vi "Coordinate_Outlier_Filtering_R2.vi"(0 "Num of Beacons":i8=5, 1 "Max Std Dev(all 5)":dbl=1.0, 5 "X in":sgl[](array[numeric]), 7 "Valid Data\nSets in":bool[](array[boolean])=[TRUE, TRUE, TRUE, TRUE, TRUE], 9 "Y in":sgl[](array[numeric]), 11 "Max Std Dev( 4 )":dbl=1.0, 13 "Max Std Dev (3)":dbl=1.0) -> (3 "Y out":sgl[](array[numeric]), 4 "Max":i32, 6 "Min Std Dev\nfor Max beacons":dbl, 8 "X out":sgl[](array[numeric]), 10 "Valid Beacons\nout":bool[](array[boolean]), 15 "Slope out":dbl)   [LabVIEW 2015]
uses:
  <vilib>/Analysis/NI_AALPro.lvlib
panel:
  out "std dev_current":dbl format="%0.6f"
  out "std dev_current 3":dbl format="%0.6f"
  out "size(s) 2":i32
  out "std dev_current 2":dbl format="%0.6f"
  out "size(s)":i32
  in  "Combo_info\nTemplate":T1={"Num Beacons"=0, "Std Dev_combo"=0.0, "Valid Data\nSets_combo"=[FALSE, FALSE, FALSE, FALSE, FALSE], "Slope combo"=0.0}
types:
  T1 = cluster{"Num Beacons":u8, "Std Dev_combo":dbl, "Valid Data\nSets_combo":bool[], "Slope combo":dbl}
  T2 = cluster{"dimension size":u8, sgl, bool[], "slope":dbl}
  T3 = cluster{"dimension size":u8, "Std Dev_combo":dbl, "Valid Data\nSets_combo":bool[], "slope":dbl}[]
  T4 = cluster{"dimension size":u8, dbl, bool[], "slope":dbl}
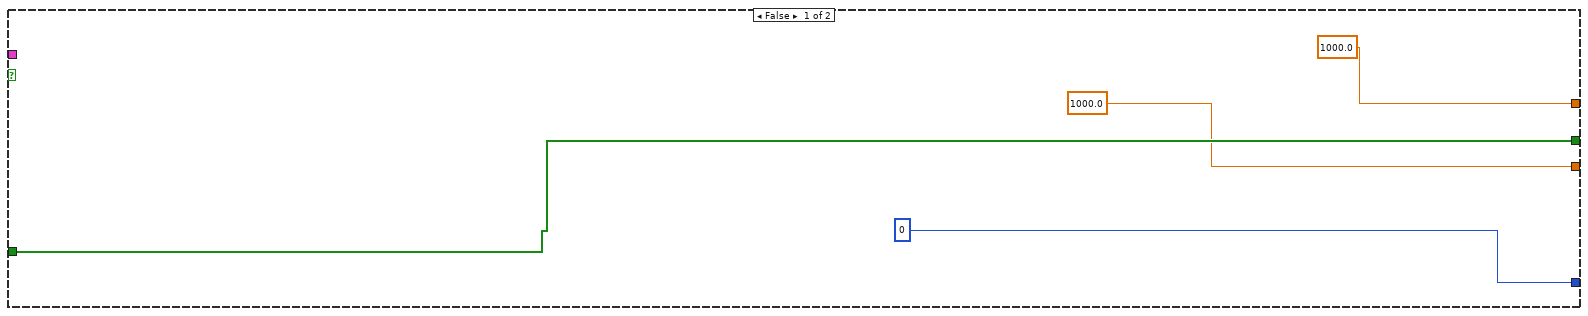
[diagram p5: hidden frame]
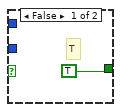
[diagram p10: hidden frame]
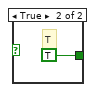
[diagram p11: hidden frame]
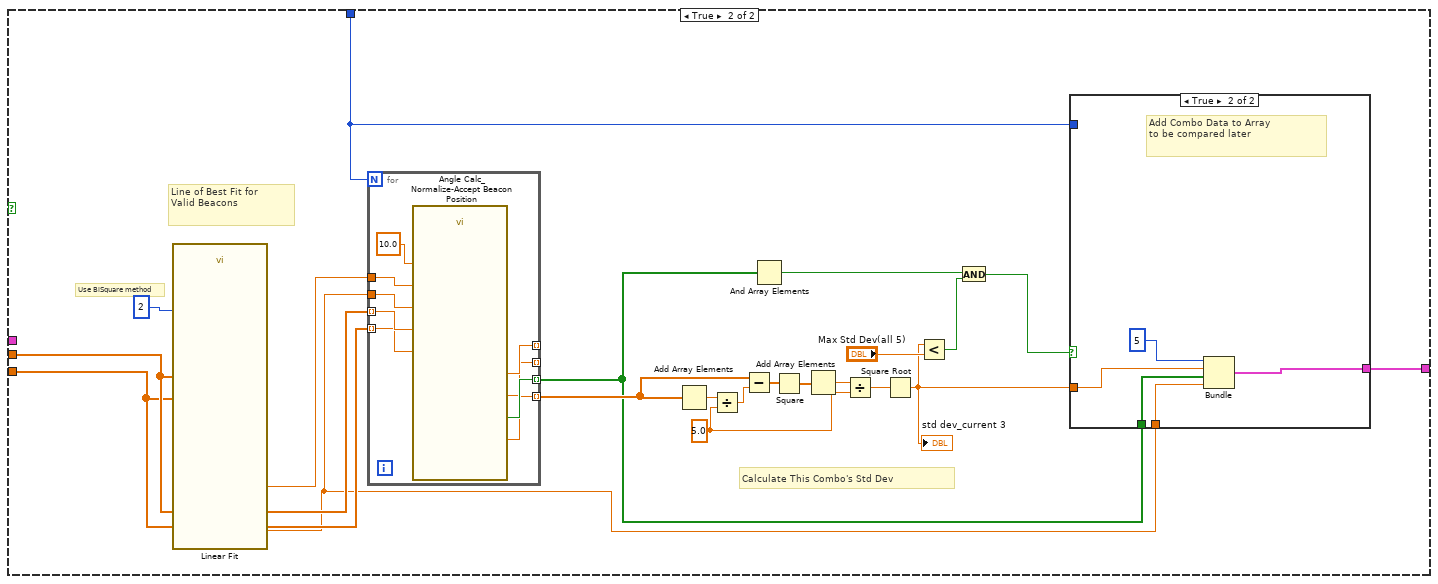
[diagram p15: hidden frame]
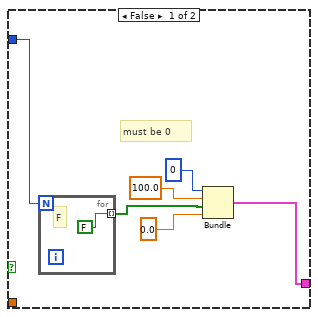
[diagram p16: hidden frame]
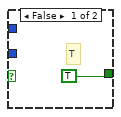
[diagram p18: hidden frame]
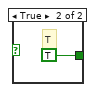
[diagram p19: hidden frame]
diagram:
  w2 = i16 2 ("y")
  # "Use BiSquare method"
  # "Line of Best Fit for\nValid Beacons"
  n1 = Boolean To (0,1)(Boolean="Valid Data\nSets in") -> (0, 1=w21:i16[])
  n2 = Add Array Elements(numeric array=w21) -> (sum=w3:i16)
  n3 = Greater?(x=w3, y=w2) -> (0:w4:bool)
  n4 = case shown="False" w4 {
    tunnel: "Combo_info\nTemplate" -> [_ w92]
    tunnel: w3 -> [_ w87]
    tunnel: "Valid Data\nSets in" -> [w24 w86]
    tunnel: [0.0 w80] -> w18
    tunnel: [0 w79] -> w17
    tunnel: [w23 w75] -> w16
    tunnel: "X in" -> [w26 w74]
    tunnel: "Y in" -> [w25 w73]
    tunnel: [w24 w72] -> w6
    tunnel: "Num of Beacons" -> [w32 w70]
    tunnel: w2 -> [w31 _]
    frame False {
      # "Use BiSquare method"
      # "Line of Best Fit for\nValid Beacons"
      # "Average"
      n5 = disable-structure shown="Disabled" {
        disable-tunnel: w26 -> [w43 _]
        disable-tunnel: w25 -> [w42 _]
        disable-tunnel: w24 -> [w41 _]
        disable-tunnel: w32 -> [w35 _]
        disable-tunnel: w31 -> [w34 _]
        frame Disabled {
          # "Grab the 2 valid coordinates"
          n6 = Initialize Array(sgl 0.0, w34) -> (w37:sgl[])
          n7 = Initialize Array(sgl 0.0, w34) -> (w38:sgl[])
          n8 = while {
            tunnel: w43 -> [w55] mode=indexing
            tunnel: w42 -> [w54] mode=indexing
            tunnel: w41 -> [w58] mode=indexing
            shift-right: [w50] -> _
            shift-left: i16 0 ("y") -> [w57]
            shift-right: [w52] -> _
            shift-left: w38 -> [w56]
            shift-right: [w51] -> _
            shift-left: w37 -> [w53]
            tunnel: w35 -> [w45]
            tunnel: w34 -> [w44]
            i -> [w46]
            stop <- w49 stop-if-true
            n9 = case shown="True" w58 {
              tunnel: w57 -> [w61 w65]
              tunnel: w56 -> [w60 w68]
              tunnel: [w61 w69] -> w50
              tunnel: w55 -> [_ w67]
              tunnel: w54 -> [_ w64]
              tunnel: w53 -> [w59 w66]
              tunnel: [w60 w63] -> w52
              tunnel: [w59 w62] -> w51
              frame False {
              }
              frame True {
                n10 = Replace Array Subset(array=w68, new element=w67, index=w65) -> (w63:sgl[])
                n11 = Replace Array Subset(array=w66, new element=w64, index=w65) -> (w62:sgl[])
                n12 = Increment(x=w65) -> (x+1=w69:i16)
              }
            }
            n13 = Greater Or Equal?(x=w46, y=w45) -> (x >= y?=w47:bool)
            n14 = Greater Or Equal?(x=w50, y=w44) -> (x >= y?=w48:bool)
            n15 = Or(x=w48, y=w47) -> (x .or. y?=w49:bool)
          }
        }
        frame Enabled {
        }
      }
      n16 = Boolean To (0,1)(Boolean=w24) -> (0, 1=w28:i16[])
      n17 = Add(x=w28, y=1e-12) -> (x+y=w30:dbl[])
      n18 = call <vilib>:"Linear Fit.vi"("Y"=w25, "X"=w26, "Weight"=w30, "method"=2) -> ("slope"=w23:dbl)  [unwired: 7 in, 4 out]
    }
    frame True {
      # "5  Beacon Combination (only 1)"
      # "4 Beacon Combinations"
      # "3 Beacon Combinations"
      n19 = Equal?(x=w87, y=5 ("dimension size")) -> (x = y?=w95:bool)
      n20 = case shown="False" w95 {
        tunnel: w74 -> [_ w320]
        tunnel: w73 -> [_ w319]
        tunnel: w70 -> [_ w304]
        tunnel: [w301 w305] -> w93
        tunnel: w92 -> [w301 _]
        frame False {
        }
        frame True {
          w303 = sgl 5.0 ("y")
          # "Calculate This Combo's Std Dev"
          # "Use BiSquare method"
          # "Line of Best Fit for\nValid Beacons"
          n21 = call <vilib>:"Linear Fit.vi"("Y"=w319, "X"=w320, "method"=2) -> ("slope"=w302:dbl, "intercept"=w321:dbl)  [unwired: 8 in, 3 out]
          n22 = for {
            N: w304 -> [_]
            tunnel: w302 -> [w342]
            tunnel: w321 -> [w341]
            tunnel: w320 -> [w340] mode=indexing
            tunnel: w319 -> [w339] mode=indexing
            tunnel: [w338] -> w306 mode=indexing
            tunnel: [w337] -> w307 mode=indexing
            tunnel: [w336] -> _ mode=indexing
            tunnel: [w335] -> _ mode=indexing
            n23 = call "Angle Calc_Normalize-Accept Beacon Position.vi"("slope"=w342, "Xin"=w340, "Deviation Threshold"=sgl 10.0 ("Deviation Threshold\n- Local Beacon Pos(*unit)"), "intercept"=w341, "Yin"=w339) -> ("Accept Beacon"=w338:bool, "Xout"=w336:sgl, "Distance"=w337:sgl, "Yout"=w335:sgl)  [unwired: 6 in, 1 out]
          }
          n24 = Add Array Elements(numeric array=w307) -> (sum=w318:sgl)
          n25 = Divide(x=w318, y=w303) -> (x/y=w317:sgl)
          n26 = Subtract(x=w307, y=w317) -> (x-y=w316:sgl[])
          n27 = And Array Elements(Boolean array=w306) -> (logical AND=w312:bool)
          n28 = Square(x=w316) -> (x^2=w308:sgl[])
          n29 = Add Array Elements(numeric array=w308) -> (sum=w314:sgl)
          n30 = Divide(x=w314, y=w303) -> (x/y=w315:sgl)
          n31 = Square Root(x=w315) -> (sqrt(x)=w310:sgl)
          "std dev_current 3" <- w310
          n32 = Less?(x=w310, y="Max Std Dev(all 5)") -> (x < y?=w311:bool)
          n33 = And(x=w312, y=w311) -> (x .and. y?=w309:bool)
          n34 = case shown="True" w309 {
            tunnel: w310 -> [_ w333]
            tunnel: w306 -> [_ w332]
            tunnel: [w325 w331] -> w305
            tunnel: w304 -> [w324 _]
            tunnel: w302 -> [_ w330]
            frame False {
              # "must be 0"
              n35 = for {
                N: w324 -> [_]
                tunnel: [FALSE] -> w326 mode=indexing
                # "F"
              }
              n36 = Bundle("dimension size"=u8 0, 100.0, w326, 0.0) -> (w325:cluster{"dimension size":u8, dbl, bool[], dbl})  [unwired: 1 in]
            }
            frame True {
              # "Add Combo Data to Array\nto be compared later"
              n37 = Bundle("dimension size"=u8 5, w333, w332, "slope"=w330) -> (w331:T2)  [unwired: 1 in]
            }
          }
        }
      }
      n38 = Build Array(w93) -> (w91:T3)
      n39 = Greater Or Equal?(x=w87, y=i16 4) -> (x >= y?=w98:bool)
      n40 = case shown="True" w98 {
        tunnel: w70 -> [_ w348]
        tunnel: w74 -> [_ w351]
        tunnel: w73 -> [_ w350]
        tunnel: w86 -> [_ w349]
        tunnel: w91 -> [w344 w347]
        tunnel: [w344 w346] -> w90
        tunnel: w70 -> [_ w345]
        frame False {
        }
        frame True {
          n41 = for {
            N: w348 -> [w355]
            shift-right: [w353] -> w346
            shift-left: w347 -> [w354]
            tunnel: w351 -> [w358]
            tunnel: w350 -> [w357]
            tunnel: w349 -> [w359]
            tunnel: w345 -> [w352]
            i -> [w356]
            n42 = for {
              N: w355 -> [w363]
              tunnel: w356 -> [w365]
              shift-right: [w361] -> w353
              shift-left: w354 -> [w362]
              tunnel: w358 -> [w367]
              tunnel: w357 -> [w366]
              tunnel: w359 -> [w368]
              tunnel: w352 -> [w360]
              i -> [w364]
              n43 = for {
                N: w363 -> [w371]
                tunnel: w368 -> [w377]
                tunnel: w367 -> [w376]
                tunnel: w366 -> [w375]
                tunnel: w365 -> [w372]
                tunnel: w364 -> [w378]
                shift-right: [w374] -> w361
                shift-left: w362 -> [w370]
                tunnel: w360 -> [w369]
                i -> [w373]
                n44 = for {
                  N: w371 -> [w388]
                  tunnel: w378 -> [w390]
                  tunnel: w377 -> [w413]
                  tunnel: w376 -> [w411]
                  tunnel: w375 -> [w410]
                  tunnel: w373 -> [w391]
                  tunnel: w372 -> [w389]
                  shift-right: [w400] -> w374
                  shift-left: w370 -> [w392]
                  tunnel: w369 -> [w379]
                  i -> [w387]
                  w393 = 4
                  # "Build Beacon Set Boolean Array\n(correlates to indexes)"
                  # "Fetch Coordinates"
                  # "Are All Indexes Different?\nAND\nDo those indexes contain valid beacons?\nAND\nIs it not a repeat combo?"
                  n45 = Greater?(x=w391, y=w390) -> (0:w383:bool)
                  n46 = Greater?(x=w390, y=w389) -> (0:w384:bool)
                  n47 = Greater?(x=w387, y=w391) -> (0:w382:bool)
                  n48 = Build Array(w389, w390, w391, w387) -> (w398:i32[])
                  n49 = for {
                    N: w393 -> [_]
                    tunnel: w398 -> [w417] mode=indexing
                    tunnel: w398 -> [w418]
                    tunnel: [w415] -> w397 mode=indexing
                    tunnel: w393 -> [w414]
                    i -> [w419]
                    n50 = for {
                      N: w414 -> [_]
                      tunnel: w419 -> [w424]
                      tunnel: w418 -> [w422] mode=indexing
                      tunnel: w417 -> [w421]
                      tunnel: [w420] -> w416 mode=indexing
                      i -> [w423]
                      n51 = Not Equal?(x=w424, y=w423) -> (x != y?=w425:bool)
                      n52 = case shown="True" w425 {
                        tunnel: w422 -> [_ w428]
                        tunnel: w421 -> [_ w427]
                        tunnel: [TRUE w429] -> w420
                        frame False {
                          # "T"
                        }
                        frame True {
                          n53 = Not Equal?(x=w427, y=w428) -> (x != y?=w429:bool)
                        }
                      }
                    }
                    n54 = And Array Elements(Boolean array=w416) -> (logical AND=w415:bool)
                  }
                  n55 = And Array Elements(Boolean array=w397) -> (logical AND=w381:bool)
                  n56 = Index Array(array=w411, index #1=w389, index #2=w390, index #3=w391, index #4=w387) -> (element #1=w409:sgl, element #2=w408:sgl, element #3=w407:sgl, element #4=w386:sgl)
                  n57 = Index Array(array=w410, index #1=w389, index #2=w390, index #3=w391, index #4=w387) -> (element #1=w406:sgl, element #2=w405:sgl, element #3=w404:sgl, element #4=w385:sgl)
                  n58 = Index Array(array=w413, index #1=w389, index #2=w390, index #3=w391, index #4=w387) -> (element #1=w396:bool, element #2=w395:bool, element #3=w394:bool, element #4=w380:bool)
                  n59 = for {
                    N: w388 -> [_]
                    tunnel: w391 -> [w440]
                    tunnel: w390 -> [w439]
                    tunnel: w389 -> [w438]
                    tunnel: [w433] -> w399 mode=indexing
                    tunnel: w387 -> [w431]
                    i -> [w432]
                    n60 = Equal?(x=w438, y=w432) -> (x = y?=w435:bool)
                    n61 = Equal?(x=w440, y=w432) -> (x = y?=w437:bool)
                    n62 = Equal?(x=w439, y=w432) -> (x = y?=w436:bool)
                    n63 = Equal?(x=w431, y=w432) -> (x = y?=w430:bool)
                    n64 = Compound Arithmetic op=OR(w437, w436, w435, w430) -> (w434:bool)
                    n65 = case shown="False" w434 {
                      tunnel: [FALSE TRUE] -> w433
                      frame False {
                        # "F"
                      }
                      frame True {
                        # "T"
                      }
                    }
                  }
                  n66 = Build Array(w409, w408, w407, w386) -> (w403:sgl[])
                  n67 = Build Array(w406, w405, w404, w385) -> (w402:sgl[])
                  n68 = Build Array(w396, w395, w394, w380) -> (w401:bool[])
                  n69 = Compound Arithmetic op=AND(w396, w395, w394, w380, w381, w382, w383, w384) -> (w412:bool)
                  n70 = case shown="True" w412 {
                    tunnel: w403 -> [_ w461]
                    tunnel: w402 -> [_ w462]
                    tunnel: w401 -> [_ w452]
                    tunnel: w392 -> [w443 w450]
                    tunnel: [w443 w448] -> w400
                    tunnel: w399 -> [_ w446]
                    tunnel: w379 -> [_ w445]
                    frame False {
                    }
                    frame True {
                      # "Calculate Distance from\nBeacon to Fitted Line"
                      # "Calculate This Combo's Std Dev"
                      # "Trim Arrays to Only Valid Beacons"
                      # "Use BiSquare method"
                      # "Line of Best Fit for\nValid Beacons"
                      # "All Indexes are Different and Beacons are Valid"
                      n71 = Initialize Array(sgl 0.0 ("element"), 4 ("dimension size")) -> (w470:sgl[])
                      n72 = for {
                        N: w445 -> [_]
                        shift-right: [w489] -> w459
                        shift-left: 0.0 -> [w490]
                        shift-right: [w488] -> w464
                        shift-left: w470 -> [w487]
                        shift-right: [w485] -> w463
                        shift-left: w470 -> [w486]
                        tunnel: w452 -> [w484] mode=indexing
                        tunnel: w461 -> [w483] mode=indexing
                        tunnel: w462 -> [w482] mode=indexing
                        n73 = case shown="True" w484 {
                          tunnel: w490 -> [w493 w500]
                          tunnel: [w493 w501] -> w489
                          tunnel: [w492 w498] -> w488
                          tunnel: w487 -> [w492 w497]
                          tunnel: w486 -> [w491 w496]
                          tunnel: [w491 w499] -> w485
                          tunnel: w483 -> [_ w495]
                          tunnel: w482 -> [_ w494]
                          frame False {
                          }
                          frame True {
                            n74 = Replace Array Subset(array=w497, new element=w495, index=w500) -> (w498:sgl[])
                            n75 = Replace Array Subset(array=w496, new element=w494, index=w500) -> (w499:sgl[])
                            n76 = Increment(x=w500) -> (x+1=w501:dbl)
                          }
                        }
                      }
                      n77 = call <vilib>:"Linear Fit.vi"("Y"=w463, "X"=w464, "method"=2) -> ("slope"=w444:dbl, "intercept"=w472:dbl)  [unwired: 8 in, 3 out]
                      n78 = for {
                        N: w445 -> [_]
                        tunnel: w472 -> [w510]
                        tunnel: w444 -> [w509]
                        tunnel: w464 -> [w508] mode=indexing
                        tunnel: w463 -> [w507] mode=indexing
                        tunnel: [w506] -> w455 mode=indexing
                        tunnel: [w505] -> _ mode=indexing
                        tunnel: [w504] -> _ mode=indexing
                        tunnel: [w503] -> w457 mode=indexing
                        n79 = call "Angle Calc_Normalize-Accept Beacon Position.vi"("slope"=w509, "Xin"=w508, "Deviation Threshold"=sgl 10.0 ("Deviation Threshold\n- Local Beacon Pos(*unit)"), "intercept"=w510, "Yin"=w507) -> ("Accept Beacon"=w506:bool, "Xout"=w505:sgl, "Distance"=w503:sgl, "Yout"=w504:sgl)  [unwired: 6 in, 1 out]
                      }
                      n80 = Add Array Elements(numeric array=w457) -> (sum=w469:sgl)
                      n81 = Divide(x=w469, y=w459) -> (x/y=w468:dbl)
                      n82 = Subtract(x=w457, y=w468) -> (x-y=w467:dbl[])
                      n83 = And Array Elements(Boolean array=w455) -> (logical AND=w454:bool)
                      n84 = Square(x=w467) -> (x^2=w456:dbl[])
                      n85 = Add Array Elements(numeric array=w456) -> (sum=w465:dbl)
                      n86 = Divide(x=w465, y=w459) -> (x/y=w466:dbl)
                      n87 = Square Root(x=w466) -> (sqrt(x)=w451:dbl)
                      "std dev_current 2" <- w451
                      n88 = Less?(x=w451, y="Max Std Dev( 4 )") -> (x < y?=w453:bool)
                      n89 = And(x=w454, y=w453) -> (x .and. y?=w449:bool)
                      n90 = case shown="True" w449 {
                        tunnel: w446 -> [_ w481]
                        tunnel: w451 -> [_ w480]
                        tunnel: w450 -> [w474 w479]
                        tunnel: [w474 w478] -> w448
                        tunnel: w444 -> [_ w475]
                        frame False {
                        }
                        frame True {
                          # "Add Combo Data to Array\nto be compared later"
                          n91 = Bundle("dimension size"=u8 4, w480, w481, "slope"=w475) -> (w476:T4)  [unwired: 1 in]
                          n92 = Build Array (concatenate)(w479, w476) -> (w478:T3)
                        }
                      }
                    }
                  }
                }
              }
            }
          }
        }
      }
      n93 = Array Size(array=w90) -> (size(s)=w96:i32)
      n94 = Decrement(x=w96) -> (x-1=w85:i32)
      "size(s) 2" <- w85
      n95 = Greater Or Equal?(x=w87, y=3 ("dimension size")) -> (x >= y?=w88:bool)
      n96 = case shown="True" w88 {
        tunnel: w70 -> [_ w156]
        tunnel: w74 -> [_ w161]
        tunnel: w73 -> [_ w160]
        tunnel: w86 -> [_ w159]
        tunnel: w90 -> [w155 w158]
        tunnel: [w155 w157] -> w82
        frame False {
        }
        frame True {
          n97 = for {
            N: w156 -> [w164]
            shift-right: [w162] -> w157
            shift-left: w158 -> [w163]
            tunnel: w161 -> [w167]
            tunnel: w160 -> [w166]
            tunnel: w159 -> [w168]
            i -> [w165]
            n98 = for {
              N: w164 -> [w171]
              tunnel: w165 -> [w173]
              shift-right: [w169] -> w162
              shift-left: w163 -> [w170]
              tunnel: w167 -> [w175]
              tunnel: w166 -> [w174]
              tunnel: w168 -> [w176]
              i -> [w172]
              n99 = for {
                N: w171 -> [w187]
                tunnel: w176 -> [w205]
                tunnel: w175 -> [w203]
                tunnel: w174 -> [w202]
                tunnel: w173 -> [w177]
                tunnel: w172 -> [w178]
                shift-right: [w188] -> w169
                shift-left: w170 -> [w189]
                i -> [w179]
                w184 = 3
                # "Build Beacon Set Boolean Array\n(correlates to indexes)"
                # "Fetch Coordinates"
                # "Are All Indexes Different?\nAND\nDo those indexes contain valid beacons?\nAND\nIs it not a repeat combo?"
                n100 = Greater?(x=w179, y=w178) -> (0:w181:bool)
                n101 = Greater?(x=w178, y=w177) -> (0:w180:bool)
                n102 = Build Array(w177, w178, w179) -> (w185:i32[])
                n103 = for {
                  N: w184 -> [_]
                  tunnel: w185 -> [w209] mode=indexing
                  tunnel: w185 -> [w210]
                  tunnel: [w207] -> w183 mode=indexing
                  tunnel: w184 -> [w206]
                  i -> [w211]
                  n104 = for {
                    N: w206 -> [_]
                    tunnel: w211 -> [w216]
                    tunnel: w210 -> [w214] mode=indexing
                    tunnel: w209 -> [w213]
                    tunnel: [w212] -> w208 mode=indexing
                    i -> [w215]
                    n105 = Not Equal?(x=w216, y=w215) -> (x != y?=w217:bool)
                    n106 = case shown="True" w217 {
                      tunnel: w214 -> [_ w220]
                      tunnel: w213 -> [_ w219]
                      tunnel: [TRUE w221] -> w212
                      frame False {
                        # "T"
                      }
                      frame True {
                        n107 = Not Equal?(x=w219, y=w220) -> (x != y?=w221:bool)
                      }
                    }
                  }
                  n108 = And Array Elements(Boolean array=w208) -> (logical AND=w207:bool)
                }
                n109 = And Array Elements(Boolean array=w183) -> (logical AND=w182:bool)
                n110 = Index Array(array=w203, index #1=w177, index #2=w178, index #3=w179) -> (element #1=w201:sgl, element #2=w200:sgl, element #3=w199:sgl)
                n111 = Index Array(array=w202, index #1=w177, index #2=w178, index #3=w179) -> (element #1=w198:sgl, element #2=w197:sgl, element #3=w196:sgl)
                n112 = for {
                  N: w187 -> [_]
                  tunnel: w179 -> [w229]
                  tunnel: w178 -> [w228]
                  tunnel: w177 -> [w227]
                  tunnel: [w222] -> w186 mode=indexing
                  i -> [w230]
                  n113 = Equal?(x=w227, y=w230) -> (x = y?=w224:bool)
                  n114 = Equal?(x=w229, y=w230) -> (x = y?=w226:bool)
                  n115 = Equal?(x=w228, y=w230) -> (x = y?=w225:bool)
                  n116 = Compound Arithmetic op=OR(w226, w225, w224) -> (w223:bool)
                  n117 = case shown="False" w223 {
                    tunnel: [FALSE TRUE] -> w222
                    frame False {
                      # "F"
                    }
                    frame True {
                      # "T"
                    }
                  }
                }
                n118 = Index Array(array=w205, index #1=w177, index #2=w178, index #3=w179) -> (element #1=w193:bool, element #2=w195:bool, element #3=w194:bool)
                n119 = Build Array(w201, w200, w199) -> (w192:sgl[])
                n120 = Build Array(w198, w197, w196) -> (w191:sgl[])
                n121 = Build Array(w193, w195, w194) -> (w190:bool[])
                n122 = Compound Arithmetic op=AND(w193, w195, w194, w182, w181, w180) -> (w204:bool)
                n123 = case shown="True" w204 {
                  tunnel: w192 -> [_ w251]
                  tunnel: w191 -> [_ w252]
                  tunnel: w190 -> [_ w242]
                  tunnel: w187 -> [_ w237]
                  tunnel: w189 -> [w233 w240]
                  tunnel: [w233 w238] -> w188
                  tunnel: w186 -> [_ w235]
                  frame False {
                  }
                  frame True {
                    # "Calculate Distance from\nBeacon to Fitted Line"
                    # "Calculate This Combo's Std Dev"
                    # "Trim Arrays to Only Valid Beacons"
                    # "Use BiSquare method"
                    # "Line of Best Fit for\nValid Beacons"
                    # "All Indexes are Different and Beacons are Valid"
                    n124 = Initialize Array(sgl 0.0 ("element"), 3 ("dimension size")) -> (w260:sgl[])
                    n125 = for {
                      N: w237 -> [_]
                      shift-right: [w279] -> w249
                      shift-left: 0.0 -> [w280]
                      shift-right: [w278] -> w254
                      shift-left: w260 -> [w277]
                      shift-right: [w275] -> w253
                      shift-left: w260 -> [w276]
                      tunnel: w242 -> [w274] mode=indexing
                      tunnel: w251 -> [w273] mode=indexing
                      tunnel: w252 -> [w272] mode=indexing
                      n126 = case shown="True" w274 {
                        tunnel: w280 -> [w283 w290]
                        tunnel: [w283 w291] -> w279
                        tunnel: [w282 w288] -> w278
                        tunnel: w277 -> [w282 w287]
                        tunnel: w276 -> [w281 w286]
                        tunnel: [w281 w289] -> w275
                        tunnel: w273 -> [_ w285]
                        tunnel: w272 -> [_ w284]
                        frame False {
                        }
                        frame True {
                          n127 = Replace Array Subset(array=w287, new element=w285, index=w290) -> (w288:sgl[])
                          n128 = Replace Array Subset(array=w286, new element=w284, index=w290) -> (w289:sgl[])
                          n129 = Increment(x=w290) -> (x+1=w291:dbl)
                        }
                      }
                    }
                    n130 = call <vilib>:"Linear Fit.vi"("Y"=w253, "X"=w254, "method"=2) -> ("slope"=w234:dbl, "intercept"=w262:dbl)  [unwired: 8 in, 3 out]
                    n131 = for {
                      N: w237 -> [_]
                      tunnel: w262 -> [w300]
                      tunnel: w234 -> [w299]
                      tunnel: w254 -> [w298] mode=indexing
                      tunnel: w253 -> [w297] mode=indexing
                      tunnel: [w296] -> w245 mode=indexing
                      tunnel: [w295] -> _ mode=indexing
                      tunnel: [w294] -> _ mode=indexing
                      tunnel: [w293] -> w247 mode=indexing
                      n132 = call "Angle Calc_Normalize-Accept Beacon Position.vi"("slope"=w299, "Xin"=w298, "Deviation Threshold"=sgl 10.0 ("Deviation Threshold\n- Local Beacon Pos(*unit)"), "intercept"=w300, "Yin"=w297) -> ("Accept Beacon"=w296:bool, "Xout"=w295:sgl, "Distance"=w293:sgl, "Yout"=w294:sgl)  [unwired: 6 in, 1 out]
                    }
                    n133 = Add Array Elements(numeric array=w247) -> (sum=w259:sgl)
                    n134 = Divide(x=w259, y=w249) -> (x/y=w258:dbl)
                    n135 = Subtract(x=w247, y=w258) -> (x-y=w257:dbl[])
                    n136 = And Array Elements(Boolean array=w245) -> (logical AND=w244:bool)
                    n137 = Square(x=w257) -> (x^2=w246:dbl[])
                    n138 = Add Array Elements(numeric array=w246) -> (sum=w255:dbl)
                    n139 = Divide(x=w255, y=w249) -> (x/y=w256:dbl)
                    n140 = Square Root(x=w256) -> (sqrt(x)=w241:dbl)
                    "std dev_current" <- w241
                    n141 = Less?(x=w241, y="Max Std Dev (3)") -> (x < y?=w243:bool)
                    n142 = And(x=w244, y=w243) -> (x .and. y?=w239:bool)
                    n143 = case shown="True" w239 {
                      tunnel: w235 -> [_ w271]
                      tunnel: w241 -> [_ w270]
                      tunnel: w240 -> [w264 w269]
                      tunnel: [w264 w268] -> w238
                      tunnel: w234 -> [_ w265]
                      frame False {
                      }
                      frame True {
                        # "Add Combo Data to Array\nto be compared later"
                        n144 = Bundle("dimension size"=u8 3, w270, w271, "slope"=w265) -> (w266:T4)  [unwired: 1 in]
                        n145 = Build Array (concatenate)(w269, w266) -> (w268:T3)
                      }
                    }
                  }
                }
              }
            }
          }
        }
      }
      n146 = Array Size(array=w82) -> (size(s)=w71:i32)
      n147 = Initialize Array(FALSE, 5 ("dimension size")) -> (w76:bool[])
      n148 = Greater Than 0?(x=w71) -> (x > 0?=w81:bool)
      n149 = case shown="True" w81 {
        tunnel: w71 -> [_ w111]
        tunnel: w82 -> [_ w113]
        tunnel: [1000.0 w110] -> w80
        tunnel: [0 w109] -> w79
        tunnel: [w102 w108] -> w72
        tunnel: w76 -> [w102 w107]
        tunnel: [1000.0 w106] -> w75
        frame False {
        }
        frame True {
          # "Pick Lowest Std Deviation\nfrom Combos with Max"
          # "Max"
          # "Find Combo with\nMax Number of Beacons"
          n150 = for {
            N: w111 -> [_]
            tunnel: w113 -> [w152] mode=indexing
            shift-right: [w150] -> w109
            shift-left: 0 -> [w148]
            n151 = Unbundle(w152) -> ("dimension size"=w149:u8)  [unwired: 3 out]
            n152 = Greater?(x=w149, y=w148) -> (0:w151:bool)
            n153 = case shown="True" w151 {
              tunnel: [w153 w154] -> w150
              tunnel: w149 -> [_ w154]
              tunnel: w148 -> [w153 _]
              frame False {
              }
              frame True {
                # "New Max"
              }
            }
          }
          n154 = Greater Than 0?(x=w109) -> (x > 0?=w112:bool)
          n155 = case shown="True" w112 {
            tunnel: w109 -> [_ w126]
            tunnel: w113 -> [_ w125]
            tunnel: w111 -> [_ w124]
            tunnel: [w116 w123] -> w110
            tunnel: [w117 w122] -> w108
            tunnel: w107 -> [w117 w121]
            tunnel: [w115 w120] -> w106
            tunnel: 1000.0 -> [w115 w119]
            tunnel: 1000.0 -> [w116 w118]
            frame False {
            }
            frame True {
              # "Min\nStd Dev"
              n156 = for {
                N: w124 -> [_]
                shift-right: [w141] -> w123
                shift-left: w118 -> [w140]
                tunnel: w125 -> [w139] mode=indexing
                tunnel: w126 -> [w138]
                shift-right: [w132] -> w122
                shift-left: w121 -> [w130]
                shift-right: [w128] -> w120
                shift-left: w119 -> [w127]
                n157 = Unbundle(w139) -> ("dimension size"=w137:u8, "Std Dev_combo"=w133:dbl, "Valid Data\nSets_combo"=w131:bool[], "slope"=w129:dbl)
                n158 = Less?(x=w133, y=w140) -> (x < y?=w134:bool)
                n159 = Equal?(x=w138, y=w137) -> (x = y?=w135:bool)
                n160 = And(x=w135, y=w134) -> (x .and. y?=w136:bool)
                n161 = case shown="True" w136 {
                  tunnel: [w144 w147] -> w141
                  tunnel: w140 -> [w144 _]
                  tunnel: w133 -> [_ w147]
                  tunnel: [w143 w146] -> w132
                  tunnel: w131 -> [_ w146]
                  tunnel: w130 -> [w143 _]
                  tunnel: [w142 w145] -> w128
                  tunnel: w129 -> [_ w145]
                  tunnel: w127 -> [w142 _]
                  frame False {
                  }
                  frame True {
                    # "New Max"
                  }
                }
              }
            }
          }
        }
      }
      n162 = Array Size(array=w82) -> (size(s)=w99:i32)
      n163 = Decrement(x=w99) -> (x-1=w84:i32)
      n164 = Subtract(x=w84, y=w85) -> (x-y=→"size(s)":i32)
    }
  }
  "Min Std Dev\nfor Max beacons" <- w18
  "Max" <- w17
  "Valid Beacons\nout" <- w6
  "Slope out" <- w16
  n165 = Boolean To (0,1)(Boolean=w6) -> (0, 1=w12:i16[])
  n166 = Add(x=w12, y=1e-12) -> (x+y=w10:dbl[])
  n167 = call <vilib>:"Linear Fit.vi"("Y"="Y in", "X"="X in", "Weight"=w10, "method"=2) -> ("slope"=w13:dbl, "intercept"=w14:dbl)  [unwired: 7 in, 3 out]
  n168 = for {
    N: "Num of Beacons" -> [_]
    tunnel: w13 -> [w517]
    tunnel: w14 -> [w516]
    tunnel: "X in" -> [w515] mode=indexing
    tunnel: "Y in" -> [w514] mode=indexing
    tunnel: [w513] -> w8 mode=indexing
    tunnel: [w512] -> w7 mode=indexing
    tunnel: w6 -> [w511] mode=indexing
    n169 = case shown="True" w511 {
      tunnel: sgl 10.0 ("Deviation Threshold\n- Local Beacon Pos(*unit)") -> [_ w526]
      tunnel: w517 -> [_ w525]
      tunnel: w516 -> [_ w524]
      tunnel: w515 -> [_ w523]
      tunnel: w514 -> [_ w522]
      tunnel: [w519 w521] -> w513
      tunnel: [w519 w520] -> w512
      frame False {
        w519 = sgl 0.0
      }
      frame True {
        n170 = call "Angle Calc_Normalize-Accept Beacon Position.vi"("slope"=w525, "Xin"=w523, "Deviation Threshold"=w526, "intercept"=w524, "Yin"=w522) -> ("Xout"=w521:sgl, "Yout"=w520:sgl)  [unwired: 6 in, 3 out]
      }
    }
  }
  "X out" <- w8
  "Y out" <- w7
